vi "hw8p2_hickey.vi"() -> ()   [LabVIEW 2014]
panel:
  out "Sum":i32
  # "First 3 runs: 15, 15, 15"
  # "Second 3 runs: 15, 15, 15"
  # "Third 3 runs: 15, 30, 45"
  # "Fourth 3 runs: 15, 30, 45"
  # "C) 0"
  # "D) The last number stored in it"
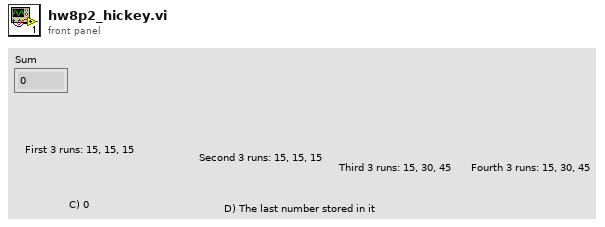
[diagram p1: front panel]
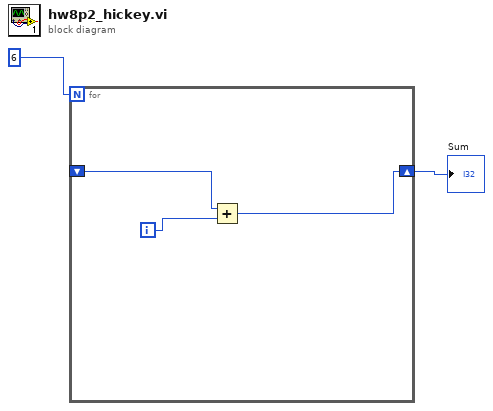
[diagram p0: block diagram]
diagram:
  n1 = for {
    N: 6 -> [_]
    shift-right: [w3] -> w1
    shift-left: _ -> [w4]
    i -> [w5]
    n2 = Add(x=w4, y=w5) -> (x+y=w3:i32)
  }
  "Sum" <- w1
